vi "Execute.vi"(6 "Index [-1]":i32=-1, 7 "Composite Object":refnum<class "CConfig Object.lvclass">, 8 "error in (no error)":errorcluster, 9 "Results":string[][](array[string]), 11 "Config Query in":refnum<class "Set Index Query.lvclass">) -> (0 "error out":errorcluster, 1 "Results":string[][](array[string]), 2 "Result":bool, 3 "Config Query out":refnum<class "Set Index Query.lvclass">, 4 "Index":i32, 5 "Composite Object":refnum<class "CConfig Object.lvclass">)   [LabVIEW 2013, in "Set Index Query.lvclass"]
doc: "Copyright 2018, Carya Automatisering, Wiebe Walstra."
uses:
  Set Index Query.lvclass
  CConfig Object.lvclass
  Set Index Query.lvclass/Set Index Query.ctl
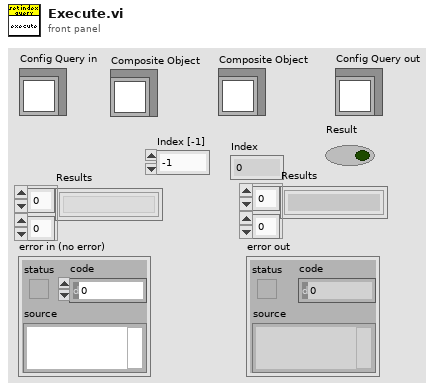
[diagram p1: front panel]
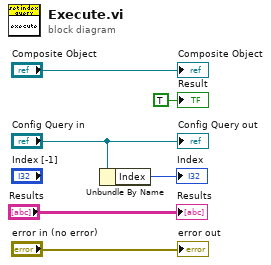
[diagram p0: block diagram]
diagram:
  n1 = Unbundle By Name("Config Query in") -> ("Index"=→"Index":i32)
  "error out" <- "error in (no error)"
  "Config Query out" <- "Config Query in"
  "Composite Object" <- "Composite Object"
  "Result" <- TRUE ("Result")
  "Results" <- "Results"
